vi "tool_Unicode_Display String Arrray (1D) Text.vi"(5 "Interpret as Unicode (T)":bool, 6 "error in":errorcluster, 8 "Value":string[](array[string]), 9 "String Array (1D) Ref":refnum<vi>) -> (0 "error out":errorcluster, 3 "String Array (1D) Ref":refnum<vi>)   [LabVIEW 2009]
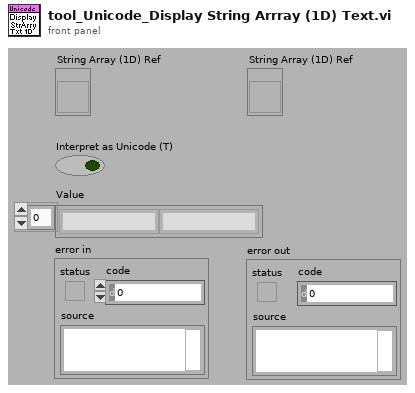
[diagram p1: front panel]
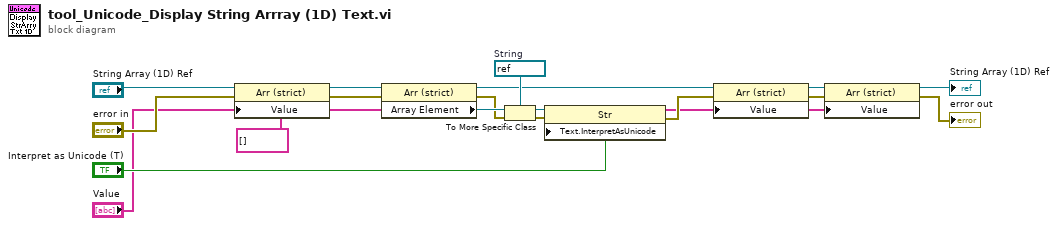
[diagram p0: block diagram]
diagram:
  w16 = refnum<vi> refnum  # String
  n1 = property class="Arr (strict)"(reference="String Array (1D) Ref", error in="error in", "Value"=string[] []) -> (reference out=w11:refnum<vi>, error out=w10:errorcluster)
  n2 = property class="Arr (strict)"(reference=w11, error in=w10) -> (reference out=w12:refnum<vi>, error out=w15:errorcluster, "Array Element"=w18:refnum<vi>)
  n3 = To More Specific Class(target class=w16, reference=w18, error in=w15) -> (specific class reference=w17:refnum<vi>, error out=w14:errorcluster)
  n4 = property class="Str"(reference=w17, error in=w14, "Text.InterpretAsUnicode"="Interpret as Unicode (T)") -> (error out=w13:errorcluster)  [unwired: 1 out]
  n5 = property class="Arr (strict)"(reference=w12, error in=w13, "Value"="Value") -> (reference out=w6:refnum<vi>, error out=w5:errorcluster)
  n6 = property class="Arr (strict)"(reference=w6, error in=w5, "Value"="Value") -> (reference out=→"String Array (1D) Ref":refnum<vi>, error out=→"error out":errorcluster)
